vi "Logging Message Loop.vi"(6 "数据通知器":refnum<notifier>, 8 "error in (no error)":errorcluster caption="错误输入（无错误）", 9 "Angle Data Queue":refnum<queue> caption="角度数据队列", 10 "Analog Data Queue":refnum<queue> caption="模拟数据队列", 11 "Message Queues":T1 caption="消息队列") -> (0 "error out":errorcluster caption="错误输出")   [LabVIEW 2015, in "Logging.lvlib"]
doc: "消息循环子VI负责处理与记录数据相关的消息。"
uses:
  Logging.lvlib
  support/Message Queue/All Message Queues.ctl
  support/Message Queue/Message Cluster.ctl
  Logging Configuration.ctl
  Logging State.ctl
  Measure/Measure Type.ctl
  <vilib>/Analysis/baseanly.llb/Mean (DBL).vi
  support/Message Queue/Enqueue Message (Single).vi
  <vilib>/Utility/file.llb/Write Delimited Spreadsheet (DBL).vi
  <vilib>/Utility/file.llb/Read Delimited Spreadsheet (DBL).vi
  <vilib>/Utility/error.llb/Error Cluster From Error Code.vi
  <vilib>/ErrorRing/Error Ring.xnode
  support/Message Queue/Message Queue.lvlib
  <vilib>/Analysis/NI_AALBase.lvlib
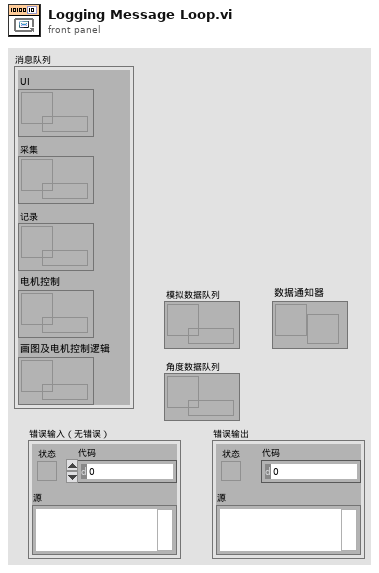
[diagram p1: front panel]
types:
  T1 = typedef "Message Queue.lvlib/All Message Queues.ctl" = cluster{"UI":refnum<queue>, "Acquisition":refnum<queue>, "Logging":refnum<queue>, "plot logic":refnum<queue>, "Action Control":refnum<queue>}
  T2 = typedef "Logging.lvlib/Logging State.ctl" = cluster{"State":enum16{"Logging", "Not Logging", "Idle"}, "Samples to Save":u32, "Force Trigger":bool}
  T3 = typedef "Logging.lvlib/Logging Configuration.ctl" = cluster{"Log File Base Path":path, "电压传感器转换率":dbl[], "电压传感器本底":dbl[], "测试模式是否需要保存数据？":bool}
  T4 = typedef "Measure Type.ctl" = enum16{"啮合", "退回", "功能", "力特性", "内泄漏", "分中", "对中"}
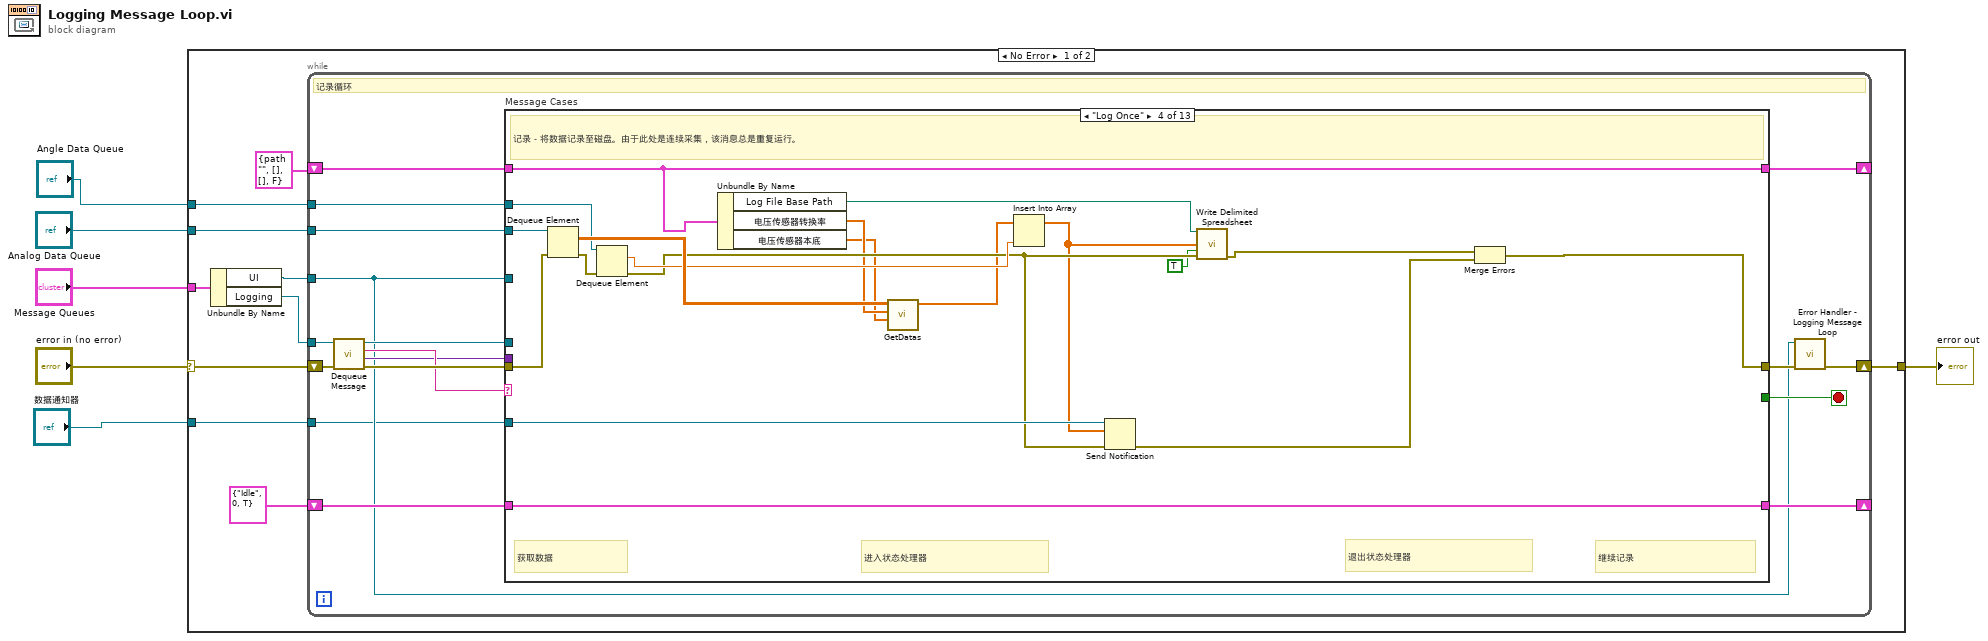
[diagram p0: block diagram]
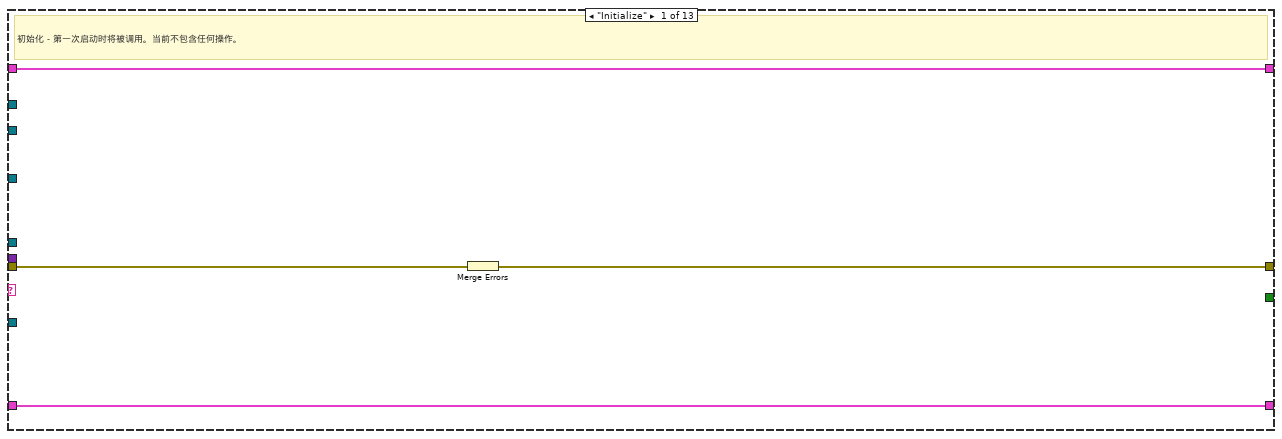
[diagram p2: hidden frame]
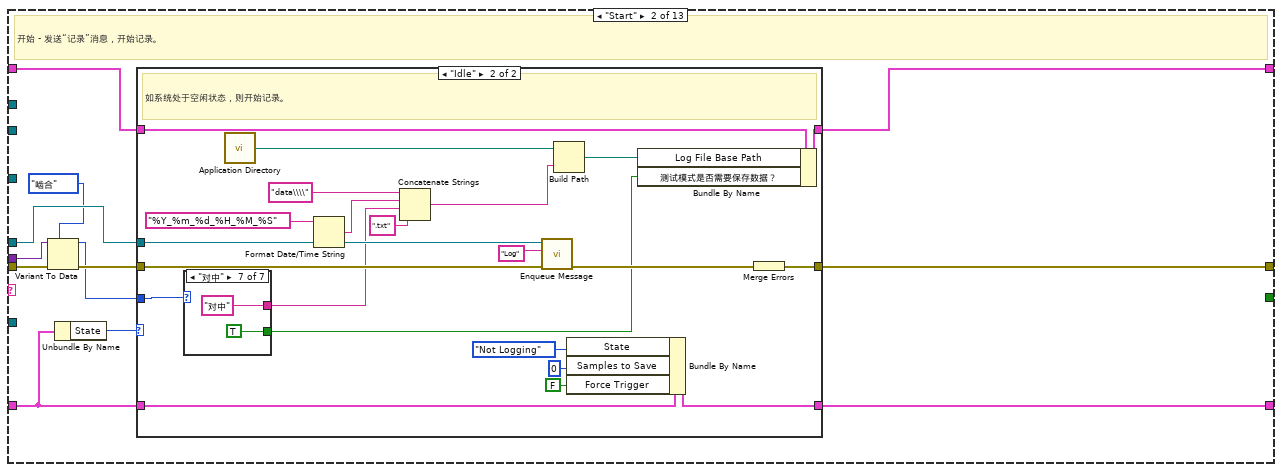
[diagram p3: hidden frame]
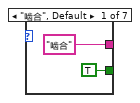
[diagram p5: hidden frame]
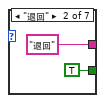
[diagram p6: hidden frame]
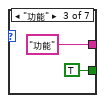
[diagram p7: hidden frame]
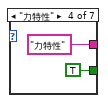
[diagram p8: hidden frame]
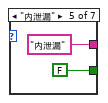
[diagram p9: hidden frame]
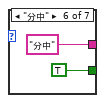
[diagram p10: hidden frame]
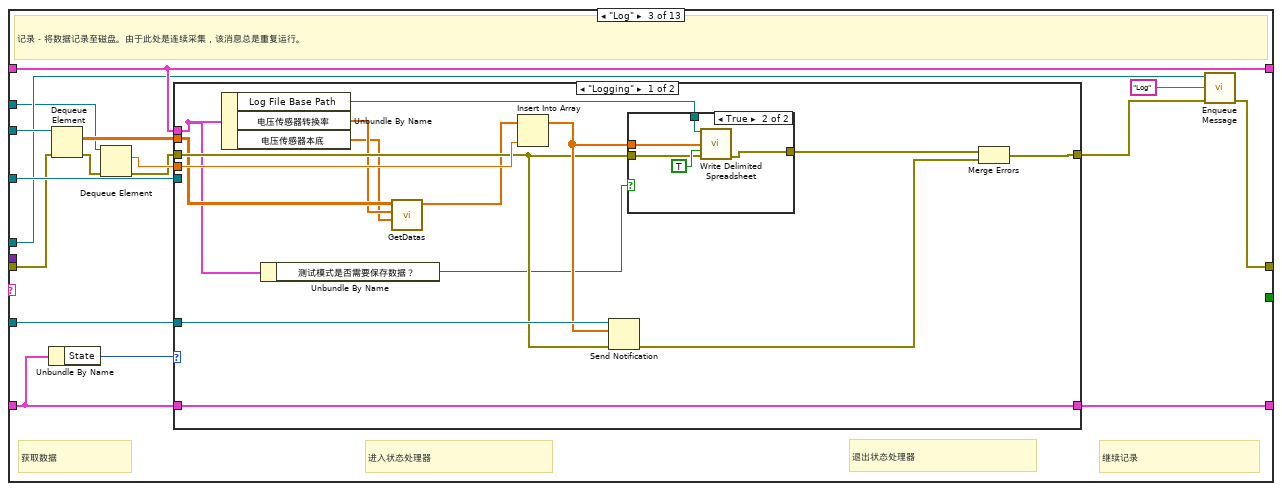
[diagram p11: hidden frame]
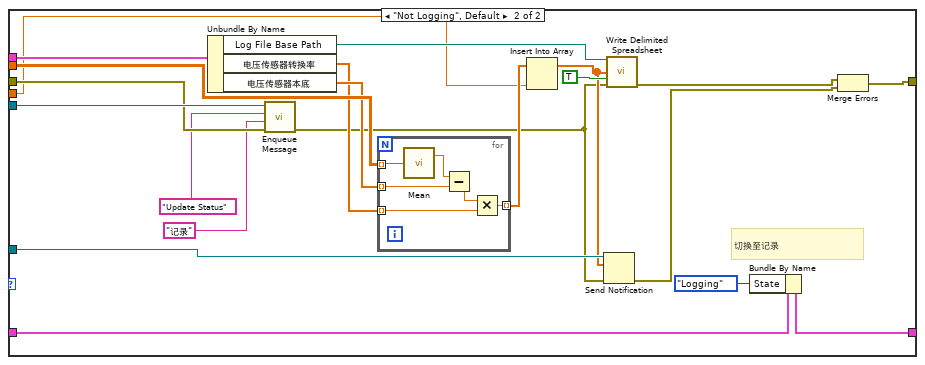
[diagram p13: hidden frame]
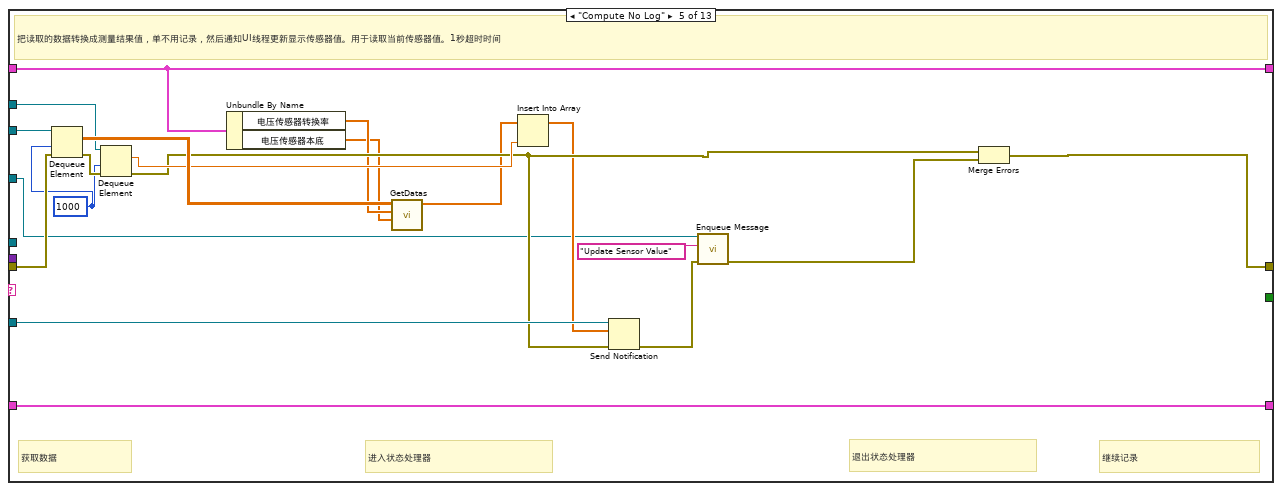
[diagram p14: hidden frame]
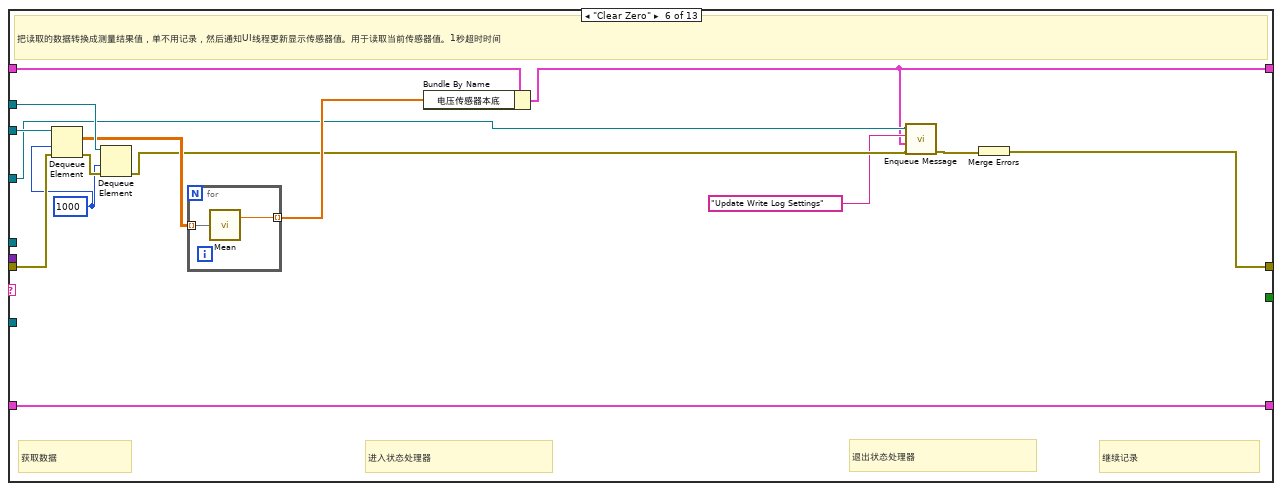
[diagram p15: hidden frame]
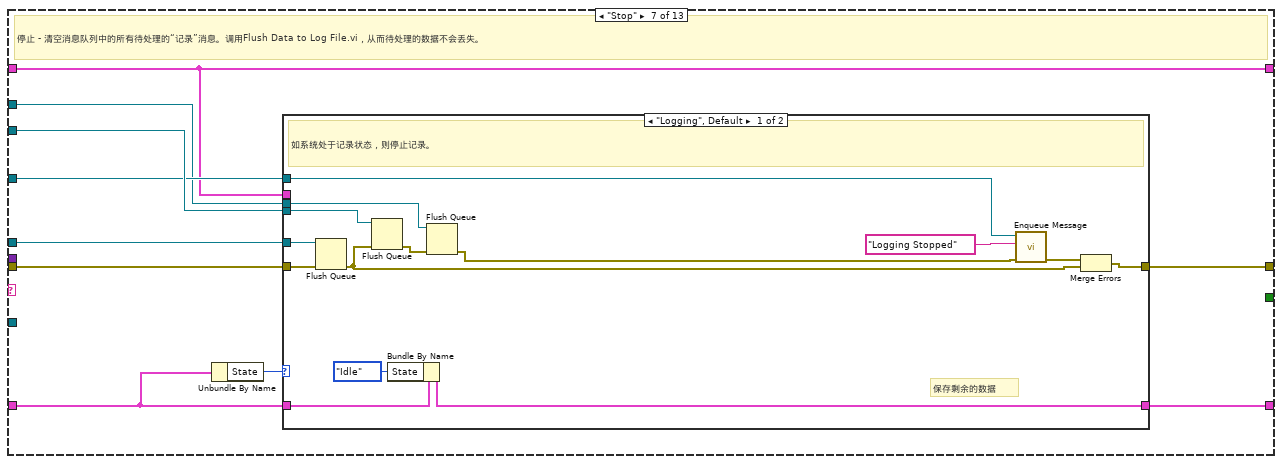
[diagram p16: hidden frame]
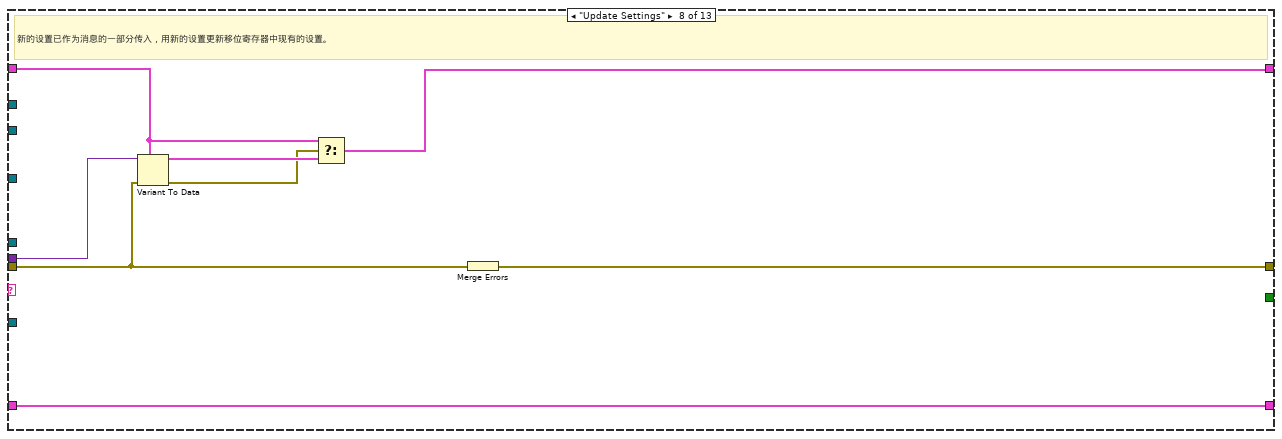
[diagram p18: hidden frame]
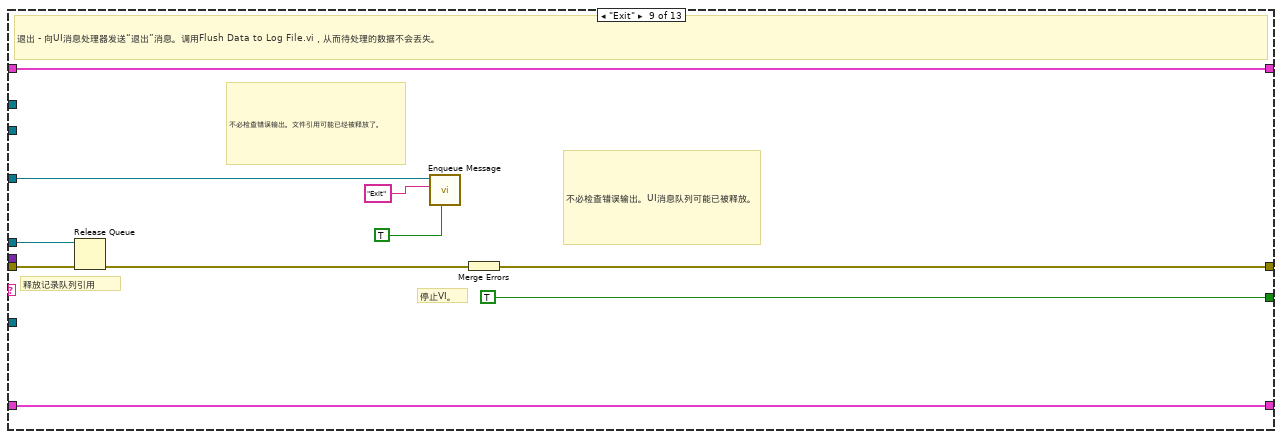
[diagram p19: hidden frame]
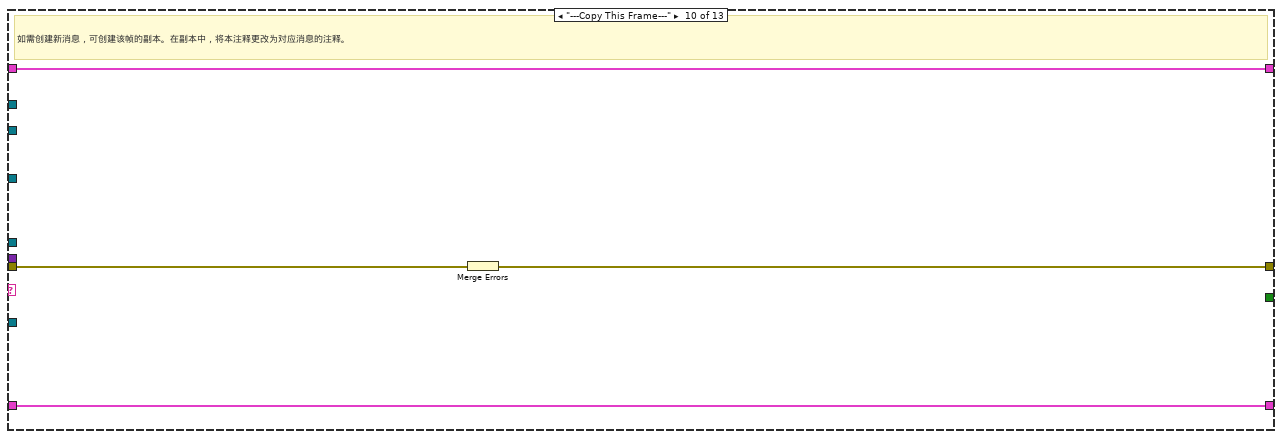
[diagram p20: hidden frame]
diagram:
  n1 = case shown="No Error" "error in (no error)" {
    selector: "error in (no error)" -> [w12 w296]
    tunnel: "Message Queues" -> [w16 _]
    tunnel: [w14 w296] -> w5
    tunnel: "Analog Data Queue" -> [w11 _]
    tunnel: "Angle Data Queue" -> [w8 _]
    tunnel: "数据通知器" -> [w7 _]
    frame No Error {
      n2 = Unbundle By Name(w16) -> ("UI"=w10:refnum<queue>, "Logging"=w15:refnum<queue>)
      n3 = while {
        tunnel: w15 -> [w25]
        shift-right: [w32] -> _
        shift-left: T3 {"Log File Base Path"=path "", "电压传感器转换率"=[], "电压传感器本底"=[], "测试模式是否需要保存数据？"=FALSE} ("Logging Configuration") -> [w33]
        shift-right: [w20] -> w14
        shift-left: w12 -> [w30]
        tunnel: w10 -> [w19]
        tunnel: w11 -> [w24]
        shift-right: [w22] -> _
        shift-left: T2 {"State"=enum."Idle", "Samples to Save"=0, "Force Trigger"=TRUE} -> [w23]
        tunnel: w8 -> [w18]
        tunnel: w7 -> [w17]
        stop <- w31 stop-if-true
        # "记录循环"
        n4 = call "Dequeue Message.vi"("error in (no error)"=w30, "Message Queue"=w25) -> ("error out"=w29:errorcluster, "Message Data"=w27:variant, "Message"=w28:string, "dup Message Queue"=w26:refnum<queue>)  [unwired: 6 in]
        n5 = case "Message Cases" shown="\"Log Once\"" w28 {
          selector: w28 -> [_ _ _ _ _ _ _ _ _ _ _ _ w285]
          tunnel: w26 -> [_ w48 w97 _ _ _ w217 _ w247 _ _ _ _]
          tunnel: w29 -> [w35 w42 w91 w165 w185 w204 w218 w237 w250 w257 w267 w282 _]
          tunnel: [w37 w49 w105 w162 w182 w202 w219 w243 w252 w255 w269 w284 w286] -> w21
          tunnel: w33 -> [w36 w47 w100 w170 w190 w199 w211 w241 w246 w256 w263 w278 w288]
          tunnel: [w36 w46 w100 w170 w190 w193 w211 w238 w246 w256 w263 w278 w288] -> w32
          tunnel: [_ _ _ _ _ _ _ _ TRUE _ _ _ _] -> w31
          tunnel: w27 -> [_ w40 _ _ _ _ _ w242 _ _ w266 w281 _]
          tunnel: w19 -> [_ _ w99 _ w176 w197 w215 _ w251 _ _ w272 _]
          tunnel: w24 -> [_ _ w98 w169 w189 w206 w216 _ _ _ _ _ _]
          tunnel: w23 -> [w34 w44 w102 w172 w192 w207 w213 w236 w244 w254 w268 w283 w287]
          tunnel: [w34 w45 w95 w172 w192 w207 w212 w236 w244 w254 w268 w283 w287] -> w22
          tunnel: w18 -> [_ _ w94 w168 w188 w205 w210 _ _ _ _ _ _]
          tunnel: w17 -> [_ _ w92 w166 w186 _ _ _ _ _ _ _ _]
          frame "Initialize" {
            # "初始化－第一次启动时将被调用。当前不包含任何操作。"
            n6 = Merge Errors(w35) -> (w37:errorcluster)
          }
          frame "Start" {
            # "开始 - 发送“记录”消息，开始记录。"
            n7 = Variant To Data(error in=w42, type=Measure_Type."啮合" ("测试类型"), Variant=w40) -> (data=w38:T4, error out=w41:errorcluster)
            n8 = Unbundle By Name(w44) -> ("State"=w43:enum16{"Logging", "Not Logging", "Idle"})
            n9 = case shown="\"Idle\"" w43 {
              tunnel: [w51 w74] -> w49
              tunnel: w48 -> [_ w73]
              tunnel: w41 -> [w51 w71]
              tunnel: w47 -> [w52 w69]
              tunnel: [w52 w68] -> w46
              tunnel: w44 -> [w50 w66]
              tunnel: [w50 w65] -> w45
              tunnel: w38 -> [_ w56]
              frame "Logging", Default {
                # "系统已经运行。忽略“开始”消息。"
              }
              frame "Idle" {
                # "如系统处于空闲状态，则开始记录。"
                n10 = case shown="\"对中\"" w56 {
                  tunnel: ["啮合" "退回" "功能" "力特性" "内泄漏" "分中" "对中"] -> w54
                  tunnel: [TRUE TRUE TRUE TRUE FALSE TRUE TRUE] -> w53
                  frame "啮合", Default {
                  }
                  frame "退回" {
                  }
                  frame "功能" {
                  }
                  frame "力特性" {
                  }
                  frame "内泄漏" {
                  }
                  frame "分中" {
                  }
                  frame "对中" {
                  }
                }
                n11 = call <vilib>:"Application Directory.vi"() -> ("Application Directory"=w59:path)
                n12 = Format Date/Time String(time format string (%c)="%Y_%m_%d_%H_%M_%S") -> (date/time string=w61:string)  [unwired: 2 in]
                n13 = Concatenate Strings("data\\\\" ("字符串"), w61, w54, ".txt" ("字符串")) -> (w60:string)
                n14 = call-poly "Enqueue Message.vi"("error in (no error)"=w71, "Message"="Log", "Message Queue"=w73) -> ("error out"=w67:errorcluster)  [unwired: 7 in, 1 out]
                n15 = Build Path(base path=w59, name or relative path=w60) -> (appended path=w57:path)
                n16 = Bundle By Name(cluster=w66, "State"=enum16{"Logging", "Not Logging"}."Not Logging", "Samples to Save"=u32 0 ("Reads to Save"), "Force Trigger"=FALSE) -> (w65:T2)
                n17 = Bundle By Name(cluster=w69, "Log File Base Path"=w57, "测试模式是否需要保存数据？"=w53) -> (w68:T3)
                n18 = Merge Errors(w67) -> (w74:errorcluster)
              }
            }
          }
          frame "Log" {
            # "退出状态处理器"
            # "继续记录"
            # "进入状态处理器"
            # "获取数据"
            # "记录－将数据记录至磁盘。由于此处是连续采集，该消息总是重复运行。"
            n19 = Unbundle By Name(w102) -> ("State"=w103:enum16{"Logging", "Not Logging", "Idle"})
            n20 = Dequeue Element(queue=w98, error in (no error)=w91) -> (element=w101:dbl[][], error out=w90:errorcluster)  [unwired: 1 in, 2 out]
            n21 = Dequeue Element(queue=w94, error in (no error)=w90) -> (element=w93:dbl, error out=w89:errorcluster)  [unwired: 1 in, 2 out]
            n22 = case shown="\"Logging\"" w103 {
              tunnel: [w120 w147] -> w95
              tunnel: w102 -> [w120 w146]
              tunnel: w101 -> [w111 w143]
              tunnel: w89 -> [w115 w142]
              tunnel: w100 -> [w107 w144]
              tunnel: w99 -> [_ w145]
              tunnel: [w113 w129] -> w96
              tunnel: w93 -> [w118 w133]
              tunnel: w92 -> [w117 w132]
              frame "Logging" {
                n23 = Unbundle By Name(w107) -> ("Log File Base Path"=w119:path, "电压传感器转换率"=w109:dbl[], "电压传感器本底"=w108:dbl[])
                n24 = Unbundle By Name(w107) -> ("测试模式是否需要保存数据？"=w106:bool)
                n25 = call "GetDatas.vi"("电压传感器本地"=w108, "电压传感器转换率"=w109, "信号数据"=w111) -> ("传感器信号"=w110:dbl[])  [unwired: 8 in]
                n26 = Insert Into Array(array=w110, new element=w118) -> (w116:dbl[])  [unwired: 1 in]
                n27 = Send Notification(notification=w116, notifier=w117, error in (no error)=w115) -> (error out=w112:errorcluster)  [unwired: 1 out]
                n28 = case shown="True" w106 {
                  tunnel: w119 -> [_ w126]
                  tunnel: w116 -> [_ w124]
                  tunnel: w115 -> [w121 w123]
                  tunnel: [w121 w122] -> w114
                  frame False {
                  }
                  frame True {
                    n29 = call-poly <vilib>:"Write Delimited Spreadsheet.vi"("file path (dialog if empty)"=w126, "1D data"=w124, "append to file? (F)"=TRUE, "error in (no error)"=w123) -> ("error out"=w122:errorcluster)  [unwired: 10 in, 1 out]
                  }
                }
                n30 = Merge Errors(w114, w112) -> (w113:errorcluster)
              }
              frame "Not Logging", Default {
                # "切换至记录"
                n31 = Unbundle By Name(w144) -> ("Log File Base Path"=w139:path, "电压传感器转换率"=w137:dbl[], "电压传感器本底"=w138:dbl[])
                n32 = call-poly "Enqueue Message.vi"("error in (no error)"=w142, "Message Data"="记录" ("Logging"), "Message"="Update Status", "Message Queue"=w145) -> ("error out"=w130:errorcluster)  [unwired: 6 in, 1 out]
                n33 = for {
                  tunnel: w143 -> [w153] mode=indexing
                  tunnel: w138 -> [w151] mode=indexing
                  tunnel: w137 -> [w149] mode=indexing
                  tunnel: [w148] -> w134 mode=indexing
                  n34 = call-poly <vilib>:"Mean.vi"("X"=w153) -> ("mean"=w152:dbl)  [unwired: 1 out]
                  n35 = Subtract(x=w152, y=w151) -> (x-y=w150:dbl)
                  n36 = Multiply(x=w150, y=w149) -> (x*y=w148:dbl)
                }
                n37 = Insert Into Array(array=w134, new element=w133) -> (w131:dbl[])  [unwired: 1 in]
                n38 = Send Notification(notification=w131, notifier=w132, error in (no error)=w130) -> (error out=w127:errorcluster)  [unwired: 1 out]
                n39 = call-poly <vilib>:"Write Delimited Spreadsheet.vi"("file path (dialog if empty)"=w139, "1D data"=w131, "append to file? (F)"=TRUE, "error in (no error)"=w130) -> ("error out"=w128:errorcluster)  [unwired: 10 in, 1 out]
                n40 = Bundle By Name(cluster=w146, "State"=enum16{"Logging", "Not Logging"}."Logging") -> (w147:T2)
                n41 = Merge Errors(w128, w127) -> (w129:errorcluster)
              }
            }
            n42 = call-poly "Enqueue Message.vi"("error in (no error)"=w96, "Message"="Log", "Message Queue"=w97) -> ("error out"=w105:errorcluster)  [unwired: 7 in, 1 out]
          }
          frame "Log Once" {
            # "退出状态处理器"
            # "继续记录"
            # "进入状态处理器"
            # "获取数据"
            # "记录－将数据记录至磁盘。由于此处是连续采集，该消息总是重复运行。"
            n43 = Dequeue Element(queue=w169, error in (no error)=w165) -> (element=w171:dbl[][], error out=w164:errorcluster)  [unwired: 1 in, 2 out]
            n44 = Dequeue Element(queue=w168, error in (no error)=w164) -> (element=w167:dbl, error out=w163:errorcluster)  [unwired: 1 in, 2 out]
            n45 = Unbundle By Name(w170) -> ("Log File Base Path"=w161:path, "电压传感器转换率"=w156:dbl[], "电压传感器本底"=w155:dbl[])
            n46 = call "GetDatas.vi"("电压传感器本地"=w155, "电压传感器转换率"=w156, "信号数据"=w171) -> ("传感器信号"=w157:dbl[])  [unwired: 8 in]
            n47 = Insert Into Array(array=w157, new element=w167) -> (w160:dbl[])  [unwired: 1 in]
            n48 = Send Notification(notification=w160, notifier=w166, error in (no error)=w163) -> (error out=w158:errorcluster)  [unwired: 1 out]
            n49 = call-poly <vilib>:"Write Delimited Spreadsheet.vi"("file path (dialog if empty)"=w161, "1D data"=w160, "append to file? (F)"=TRUE, "error in (no error)"=w163) -> ("error out"=w159:errorcluster)  [unwired: 10 in, 1 out]
            n50 = Merge Errors(w159, w158) -> (w162:errorcluster)
          }
          frame "Compute No Log" {
            w177 = 1000 ("timeout in ms (-1)")
            # "退出状态处理器"
            # "继续记录"
            # "进入状态处理器"
            # "获取数据"
            # "把读取的数据转换成测量结果值，单不用记录，然后通知UI线程更新显示传感器值。用于读取当前传感器值。1秒超时时间"
            n51 = Dequeue Element(queue=w189, timeout in ms (-1)=w177, error in (no error)=w185) -> (element=w191:dbl[][], error out=w184:errorcluster)  [unwired: 2 out]
            n52 = Dequeue Element(queue=w188, timeout in ms (-1)=w177, error in (no error)=w184) -> (element=w187:dbl, error out=w183:errorcluster)  [unwired: 2 out]
            n53 = Unbundle By Name(w190) -> ("电压传感器转换率"=w179:dbl[], "电压传感器本底"=w178:dbl[])
            n54 = call "GetDatas.vi"("电压传感器本地"=w178, "电压传感器转换率"=w179, "信号数据"=w191) -> ("传感器信号"=w180:dbl[])  [unwired: 8 in]
            n55 = Insert Into Array(array=w180, new element=w187) -> (w181:dbl[])  [unwired: 1 in]
            n56 = Send Notification(notification=w181, notifier=w186, error in (no error)=w183) -> (error out=w174:errorcluster)  [unwired: 1 out]
            n57 = call-poly "Enqueue Message.vi"("error in (no error)"=w174, "Message"="Update Sensor Value", "Message Queue"=w176) -> ("error out"=w173:errorcluster)  [unwired: 7 in, 1 out]
            n58 = Merge Errors(w183, w173) -> (w182:errorcluster)
          }
          frame "Clear Zero" {
            w201 = 1000 ("timeout in ms (-1)")
            # "退出状态处理器"
            # "继续记录"
            # "进入状态处理器"
            # "获取数据"
            # "把读取的数据转换成测量结果值，单不用记录，然后通知UI线程更新显示传感器值。用于读取当前传感器值。1秒超时时间"
            n59 = Dequeue Element(queue=w206, timeout in ms (-1)=w201, error in (no error)=w204) -> (element=w200:dbl[][], error out=w203:errorcluster)  [unwired: 2 out]
            n60 = Dequeue Element(queue=w205, timeout in ms (-1)=w201, error in (no error)=w203) -> (error out=w196:errorcluster)  [unwired: 3 out]
            n61 = for {
              tunnel: w200 -> [w209] mode=indexing
              tunnel: [w208] -> w198 mode=indexing
              n62 = call-poly <vilib>:"Mean.vi"("X"=w209) -> ("mean"=w208:dbl)  [unwired: 1 out]
            }
            n63 = Bundle By Name(cluster=w199, "电压传感器本底"=w198) -> (w193:T3)
            n64 = call-poly "Enqueue Message.vi"("error in (no error)"=w196, "Message Data"=w193, "Message"="Update Write Log Settings", "Message Queue"=w197) -> ("error out"=w195:errorcluster)  [unwired: 6 in, 1 out]
            n65 = Merge Errors(w195) -> (w202:errorcluster)
          }
          frame "Stop" {
            # "停止 - 清空消息队列中的所有待处理的“记录”消息。调用Flush Data to Log File.vi，从而待处理的数据不会丢失。"
            n66 = Unbundle By Name(w213) -> ("State"=w214:enum16{"Logging", "Not Logging", "Idle"})
            n67 = case shown="\"Logging\", Default" w214 {
              tunnel: [w233 w235] -> w219
              tunnel: w218 -> [w232 w235]
              tunnel: w217 -> [w231 _]
              tunnel: w211 -> [_ _]
              tunnel: w216 -> [w224 _]
              tunnel: w215 -> [w229 _]
              tunnel: w213 -> [w227 w234]
              tunnel: [w226 w234] -> w212
              tunnel: w210 -> [w221 _]
              frame "Logging", Default {
                # "保存剩余的数据"
                # "如系统处于记录状态，则停止记录。"
                n68 = Flush Queue(queue=w231, error in (no error)=w232) -> (error out=w223:errorcluster)  [unwired: 2 out]
                n69 = Flush Queue(queue=w224, error in (no error)=w223) -> (error out=w222:errorcluster)  [unwired: 2 out]
                n70 = Bundle By Name(cluster=w227, "State"=enum16{"Logging", "Not Logging", "Idle"}."Idle") -> (w226:T2)
                n71 = Flush Queue(queue=w221, error in (no error)=w222) -> (error out=w220:errorcluster)  [unwired: 2 out]
                n72 = call-poly "Enqueue Message.vi"("error in (no error)"=w220, "Message"="Logging Stopped", "Message Queue"=w229) -> ("error out"=w230:errorcluster)  [unwired: 7 in, 1 out]
                n73 = Merge Errors(w230, w223) -> (w233:errorcluster)
              }
              frame "Idle" {
                # "系统已处于空闲状态。忽略“停止”消息。"
              }
            }
          }
          frame "Update Settings" {
            # "新的设置已作为消息的一部分传入，用新的设置更新移位寄存器中现有的设置。"
            n74 = Variant To Data(error in=w237, type=w241, Variant=w242) -> (data=w240:T3, error out=w239:errorcluster)
            n75 = Select(t=w241, s=w239, f=w240) -> (s? t:f=w238:T3)
            n76 = Merge Errors(w237) -> (w243:errorcluster)
          }
          frame "Exit" {
            # "不必检查错误输出。文件引用可能已经被释放了。"
            # "释放记录队列引用"
            # "不必检查错误输出。UI消息队列可能已被释放。"
            # "停止VI。"
            # "退出 - 向UI消息处理器发送“退出”消息。调用Flush Data to Log File.vi，从而待处理的数据不会丢失。"
            n77 = Release Queue(queue=w247, error in (no error)=w250) -> (error out=w245:errorcluster)  [unwired: 1 in, 2 out]
            n78 = call-poly "Enqueue Message.vi"("Priority Message? (F)"=TRUE, "Message"="Exit", "Message Queue"=w251) -> ()  [unwired: 7 in, 2 out]
            n79 = Merge Errors(w245) -> (w252:errorcluster)
          }
          frame "---Copy This Frame---" {
            # "如需创建新消息，可创建该帧的副本。在副本中，将本注释更改为对应消息的注释。"
            n80 = Merge Errors(w257) -> (w255:errorcluster)
          }
          frame "Calculate" {
            # "如需创建新消息，可创建该帧的副本。在副本中，将本注释更改为对应消息的注释。"
            n81 = Unbundle By Name(w263) -> ("Log File Base Path"=w262:path)
            n82 = Variant To Data(error in=w267, type=Measure_Type."啮合" ("计算类型"), Variant=w266) -> (data=w259:T4, error out=w264:errorcluster)
            n83 = call-poly <vilib>:"Read Delimited Spreadsheet.vi"("file path (dialog if empty)"=w262, "error in (no error)"=w264) -> ("all rows"=w260:dbl[][], "error out"=w261:errorcluster)  [unwired: 8 in, 4 out]
            n84 = call "计算类型执行.vi"("error in (no error)"=w261, "信号数据"=w260, "计算类型"=w259) -> ("error out"=w258:errorcluster)  [unwired: 8 in]
            n85 = Merge Errors(w258) -> (w269:errorcluster)
          }
          frame "Calculate分中" {
            # "如需创建新消息，可创建该帧的副本。在副本中，将本注释更改为对应消息的注释。"
            n86 = Unbundle By Name(w278) -> ("Log File Base Path"=w277:path)
            n87 = Variant To Data(error in=w282, type=Measure_Type."分中" ("计算类型"), Variant=w281) -> (error out=w279:errorcluster)  [unwired: 1 out]
            n88 = call-poly <vilib>:"Read Delimited Spreadsheet.vi"("file path (dialog if empty)"=w277, "error in (no error)"=w279) -> ("all rows"=w275:dbl[][], "error out"=w276:errorcluster)  [unwired: 8 in, 4 out]
            n89 = call "分中.vi"("error in (no error)"=w276, "信号数据"=w275) -> ("error out"=w274:errorcluster, "分中角度"=w271:dbl)  [unwired: 8 in]
            n90 = call-poly "Enqueue Message.vi"("error in (no error)"=w274, "Message Data"=w271, "Message"="分中_更新停止角度", "Message Queue"=w272) -> ("error out"=w273:errorcluster)  [unwired: 6 in, 1 out]
            n91 = Merge Errors(w273) -> (w284:errorcluster)
          }
          frame Default {
            # "如得到的消息未经任何分支定义，则运行“默认”分支。输出程序错误。"
            n92 = xnode "Error Ring"("parameter 0"=w285) -> ("error out"=w286:errorcluster)
          }
        }
        n93 = call "Error Handler - Logging Message Loop.vi"("error in (no error)"=w21, "Message Queue"=w19) -> ("dup error in"=w20:errorcluster)  [unwired: 8 in, 1 out]
      }
    }
    frame Error {
    }
  }
  "error out" <- w5
